vi "extract_ref_temp.vi"(6 "name":string, 8 "name_array":string[](array[string]), 9 "value_array":dbl[](array[numeric]), 11 "time":timestamp) -> (0 "temp_K":dbl, 1 "temp_F":dbl, 2 "temp_array":dbl[](array[numeric]), 3 "waveform_array":waveform(dbl)[](array[waveform])=[{"t0"=timestamp(0 s since 1904-01-01), "dt"=1.0, "Y"=[]}, {"t0"=timestamp(3732035173.078092 s since 1904-01-01), "dt"=1.0, "Y"=[302.8589782714844], "attributes"=variant("NI_ChannelName"=variant(string "T1"))}])   [LabVIEW 2019]
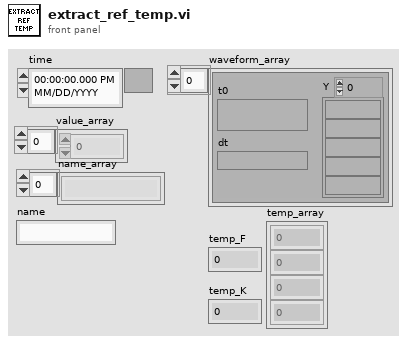
[diagram p1: front panel]
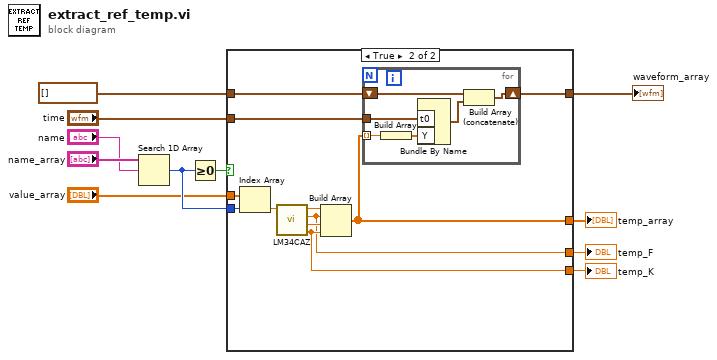
[diagram p0: block diagram]
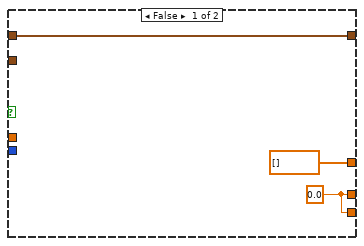
[diagram p2: hidden frame]
diagram:
  n1 = Search 1D Array(1D array="name_array", element="name") -> (index of element=w8:i32)  [unwired: 1 in]
  n2 = Greater Or Equal To 0?(x=w8) -> (x >= 0?=w9:bool)
  n3 = case shown="True" w9 {
    tunnel: w8 -> [_ w25]
    tunnel: "value_array" -> [_ w24]
    tunnel: waveform(dbl)[] [] -> [w14 w20]
    tunnel: "time" -> [_ w19]
    tunnel: [w14 w18] -> w4
    tunnel: [dbl[] [] w17] -> w3
    tunnel: [w12 w16] -> w2
    tunnel: [w12 w15] -> w1
    frame False {
      w12 = 0.0 ("CJC (K)")
    }
    frame True {
      n4 = Index Array(array=w24, index=w25) -> (element=w23:dbl)
      n5 = call "LM34CAZ.vi"("voltage"=w23) -> ("CJC (K)"=w16:dbl, "CJC (C)"=w21:dbl, "CJC (F)"=w15:dbl, "CJC (V)"=w22:dbl)  [unwired: 7 in]
      n6 = Build Array(w22, w15, w21, w16) -> (w17:dbl[])
      n7 = for {
        tunnel: w19 -> [w29]
        tunnel: w17 -> [w27] mode=indexing
        shift-right: [w28] -> w18
        shift-left: w20 -> [w31]
        n8 = Build Array(w27) -> (w30:dbl[])
        n9 = Bundle By Name("t0"=w29, "Y"=w30) -> (w26:waveform(dbl))  [unwired: 1 in]
        n10 = Build Array (concatenate)(w31, w26) -> (w28:waveform(dbl)[])
      }
    }
  }
  "waveform_array" <- w4
  "temp_array" <- w3
  "temp_K" <- w2
  "temp_F" <- w1
